vi "Log Data to File.vi"(7 "WriteLogFile (T)":bool=TRUE, 8 "error in (no error)":errorcluster, 10 "Path":path) -> (0 "error out":errorcluster, 2 "Path out":path)   [LabVIEW 2017, in "LogEngine.lvclass"]
doc: "Developed by Kevin Thompson\nkevin@thompsonengineering.net\n\nCopyright 2018-2020\nThompson Engineering, LLC"
uses:
  LogEngine.lvclass
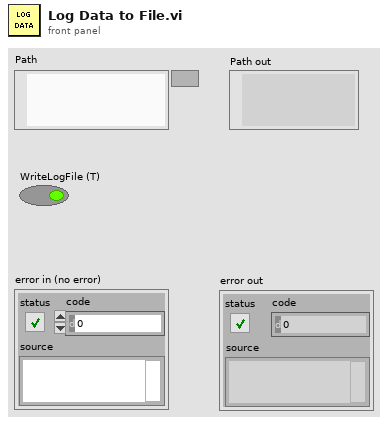
[diagram p1: front panel]
types:
  T1 = typedef "TD MeasData--cluster.ctl" = cluster{"Timestamp":timestamp, "StepNumber":i32, "WeldCurrentSP_A":dbl, "VoltageDyn_V":dbl, "CurrentDyn_A":dbl, "VSPSum_V":dbl, "VoltageError_V":dbl, "P val":dbl, "D val":dbl, "I val":dbl, "ID Error":dbl, "TotalCtlrGain_V":dbl, "TotalMove_mil":dbl, "AVCLockout":bool}
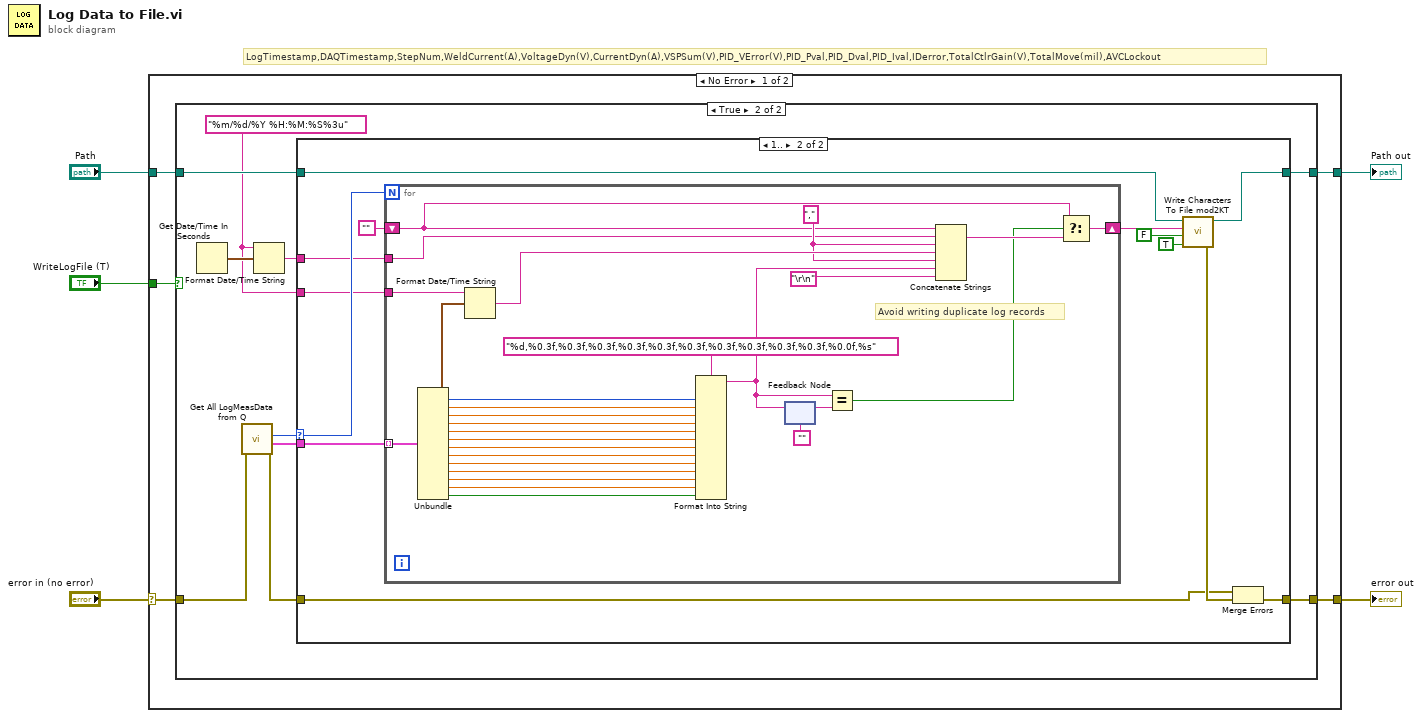
[diagram p0: block diagram]
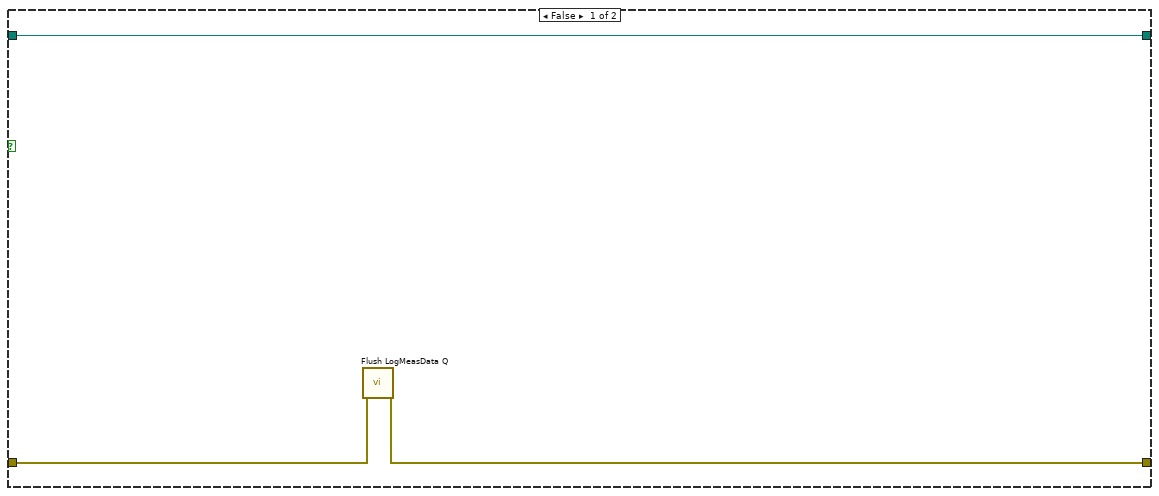
[diagram p2: hidden frame]
diagram:
  # "LogTimestamp,DAQTimestamp,StepNum,WeldCurrent(A),VoltageDyn(V),CurrentDyn(A),VSPSum(V),PID_VError(V),PID_Pval,PID_Dval,PID_Ival,IDerror,TotalCtlrGain(V),TotalMove(mil),AVCLockout"
  n1 = case shown="No Error" "error in (no error)" {
    selector: "error in (no error)" -> [w10 w68]
    tunnel: [w7 w68] -> w4
    tunnel: "Path" -> [w9 w67]
    tunnel: [w8 w67] -> w2
    tunnel: "WriteLogFile (T)" -> [w6 _]
    frame No Error {
      n2 = case shown="True" w6 {
        tunnel: w10 -> [w13 w23]
        tunnel: w9 -> [w11 w20]
        tunnel: [w11 w19] -> w8
        tunnel: [w12 w18] -> w7
        frame False {
          n3 = call "Flush LogMeasData Q.vi"("error in (no error)"=w13) -> ("error out"=w12:errorcluster)  [unwired: 8 in, 2 out]
        }
        frame True {
          w14 = "%m/%d/%Y %H:%M:%S%3u"
          n4 = Get Date/Time In Seconds() -> (seconds since 1Jan1904=w16:timestamp)
          n5 = call "Get All LogMeasData from Q.vi"("error in (no error)"=w23) -> ("error out"=w17:errorcluster, "MeasData[] out"=w21:T1[], "NumElements"=w22:i32)  [unwired: 7 in, 1 out]
          n6 = Format Date/Time String(time format string (%c)=w14, seconds (now)=w16) -> (date/time string=w15:string)  [unwired: 1 in]
          n7 = case shown="1.." w22 {
            selector: w22 -> [_ w38]
            tunnel: w21 -> [_ w37]
            tunnel: w20 -> [w25 w34]
            tunnel: [w25 w31] -> w19
            tunnel: [w24 w29] -> w18
            tunnel: w17 -> [w24 w28]
            tunnel: w15 -> [_ w27]
            tunnel: w14 -> [_ w26]
            frame ..0 {
            }
            frame 1.. {
              n8 = for {
                N: w38 -> [_]
                tunnel: w37 -> [w66] mode=indexing
                shift-right: [w43] -> w35
                shift-left: "" -> [w44]
                tunnel: w27 -> [w56]
                tunnel: w26 -> [w46]
                w58 = ","
                # "Avoid writing duplicate log records"
                n9 = Unbundle(w66) -> ("Timestamp"=w65:timestamp, "StepNumber"=w64:i32, "WeldCurrentSP_A"=w63:dbl, "VoltageDyn_V"=w62:dbl, "CurrentDyn_A"=w61:dbl, "VSPSum_V"=w55:dbl, "VoltageError_V"=w54:dbl, "P val"=w53:dbl, "D val"=w52:dbl, "I val"=w51:dbl, "ID Error"=w50:dbl, "TotalCtlrGain_V"=w49:dbl, "TotalMove_mil"=w48:dbl, "AVCLockout"=w47:bool)
                n10 = Format Date/Time String(time format string (%c)=w46, seconds (now)=w65) -> (date/time string=w59:string)  [unwired: 1 in]
                n11 = Format Into String(format string="%d,%0.3f,%0.3f,%0.3f,%0.3f,%0.3f,%0.3f,%0.3f,%0.3f,%0.3f,%0.3f,%0.0f,%s", w64, w63, w62, w61, w55, w54, w53, w52, w51, w50, w49, w48, w47) -> (resulting string=w40:string)  [unwired: 2 in, 1 out]
                n12 = feedback-in #1(w40) -> ()
                n13 = feedback #1("") -> (w41:string)
                n14 = Equal?(x=w40, y=w41) -> (x = y?=w39:bool)
                n15 = Concatenate Strings(w44, w56, w58, w59, w58, w40, "\r\n") -> (w45:string)
                n16 = Select(t=w44, s=w39, f=w45) -> (s? t:f=w43:string)
              }
              n17 = call <vilib>:"Write Characters To File mod2KT.vi"("append to file? (new file:F)"=TRUE, "advisory dialog? (display:T)"=FALSE, "character string"=w35, "file path (dialog if empty)"=w34) -> ("error out"=w30:errorcluster, "new file path (Not A Path if cancelled)"=w31:path)  [unwired: 2 in]
              n18 = Merge Errors(w28, w30) -> (w29:errorcluster)
            }
          }
        }
      }
    }
    frame Error {
    }
  }
  "error out" <- w4
  "Path out" <- w2
